vi "SVPO Envelope Detection.vi"   [LabVIEW 2017, in "SoundVib_FaultAnalysis.lvlib"]
doc: "Extracts the modulating signal, or envelope signal, from an amplitude-modulated signal. You can use the envelope detection technique to identify the mechanical faults that have amplitude-modulating effect on the vibration signal of a machine. Use this VI on embedded targets that have limited computational resources. Wire data to the <B>scaled signal [EU]</B> input to determine the polymorphic instance to use or manually select the instance."
uses:
  <vilib>/addons/Sound and Vibration/Order Analysis/Fault Analysis/SoundVib_FaultAnalysis.lvlib
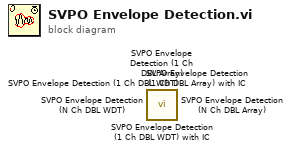
[diagram p0: block diagram]
diagram:
  n1 = call <vilib>:"SVPO Envelope Detection (1 Ch DBL WDT) with IC.vi"() -> ()  [unwired: 14 in, 2 out]
  n2 = call <vilib>:"SVPO Envelope Detection (1 Ch DBL Array) with IC.vi"() -> ()  [unwired: 13 in, 3 out]
  n3 = call <vilib>:"SVPO Envelope Detection (N Ch DBL WDT).vi"() -> ()  [unwired: 15 in, 1 out]
  n4 = call <vilib>:"SVPO Envelope Detection (N Ch DBL Array).vi"() -> ()  [unwired: 14 in, 2 out]
  n5 = call <vilib>:"SVPO Envelope Detection (1 Ch DBL WDT).vi"() -> ()  [unwired: 15 in, 1 out]
  n6 = call <vilib>:"SVPO Envelope Detection (1 Ch DBL Array).vi"() -> ()  [unwired: 14 in, 2 out]
